vi "TSM Relay Connections to Configuration_v2.vi"(0 "TSM Context":T6, 5 "Relay/Action Connections":T4[](array[typedef]) {"Relay Action" items=["Open Relay"=20, "Close Relay"=21]}, 9 "TSM Site Numbers":i32[](array[numeric]), 11 "error in":errorcluster) -> (4 "TSM Relay Configuration":T1 {"SSC Relay with Action"."Relay Action" items=["Open Relay"=20, "Close Relay"=21]}, 15 "error out":errorcluster)   [LabVIEW 2019]
doc: "Populates the TSM Relay Configuration cluster for the selected relay/action connections. This VI can be used to implement a relay configuration (set of mappings between relays and positions) within a test code module. \n\nUse this VI in place of TSM Relay Conections to Configuration VI when optimizing for test time - this allows users to call Get Site Numbers only once in their code module and reduce the number of TSM context calls."
uses:
  <vilib>/NI_TestStand_SemiconductorModule/NI_TestStand_Semiconductor_Module.lvlibp/PinMap/General/SemiconductorModuleContext.ctl
  Pin Map/TSM Relay to Action Map.ctl
  <vilib>/NI_TestStand_SemiconductorModule/NI_TestStand_Semiconductor_Module.lvlibp/1abvi3w/instr.lib/niSwitch/niswitch.llb/niSwitch Relay Action.ctl
  SubVIs/TSM Relay Config.ctl
  <vilib>/NI_TestStand_SemiconductorModule/NI_TestStand_Semiconductor_Module.lvlibp/PinMap/PinQueryContext/MultiplePinMultipleSessionQueryContext/MultiplePinMultipleSessionQueryContext.lvclass
  SSC/SSC Relay.ctl
  <instrlib>/niSwitch/niSwitch.llb/niSwitch Relay Action.ctl
  <vilib>/NI_TestStand_SemiconductorModule/NI_TestStand_Semiconductor_Module.lvlibp
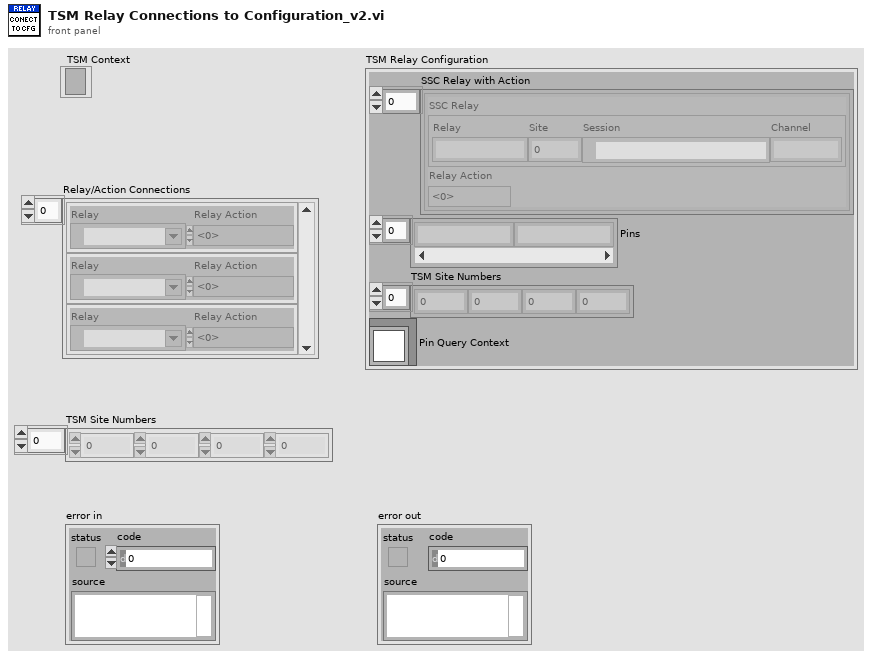
[diagram p1: front panel]
types:
  T1 = typedef "TSM Relay Config.ctl" = cluster{"SSC Relay with Action":cluster{"SSC Relay":T2, "Relay Action":T3}[], "Pins":string[], "TSM Site Numbers":i32[], "Pin Query Context":refnum<class "MultiplePinMultipleSessionQueryContext.lvclass">}
  T2 = typedef "SSC Relay.ctl" = cluster{"Relay":string, "Site":i32, "Session":refnum<k15>, "Channel":string}
  T3 = typedef "niSwitch Relay Action.ctl" = i32
  T4 = typedef "TSM Relay to Action Map.ctl" = cluster{"Relay":tag, "Relay Action":T5}
  T5 = typedef "NI_TestStand_Semiconductor_Module.lvlibp/niSwitch Relay Action.ctl" = i32
  T6 = typedef "NI_TestStand_Semiconductor_Module.lvlibp/SemiconductorModuleContext.ctl" = refnum<k7>
  T7 = typedef "TSM SSC Relay.ctl" = cluster{"TSM context":T6, "Pin Query Context":refnum<class "MultiplePinMultipleSessionQueryContext.lvclass">, "TSM Site Numbers":i32[], "SSC Relay":T2[], "Unfiltered Pins":string[], "Filtered Pins":string[], "Filtered Pins Info":T8}
  T8 = typedef "TSM Filtered Pins Info.ctl" = cluster{"Unfiltered Pins Count":i32, "Locations":i32[], "Lengths":i32[]}
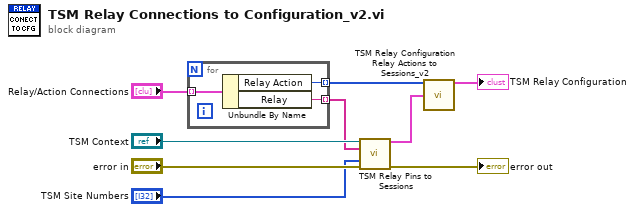
[diagram p0: block diagram]
diagram:
  n1 = for {
    tunnel: "Relay/Action Connections" -> [w11] mode=indexing
    tunnel: [w12] -> w2 mode=indexing
    tunnel: [w10] -> w5 mode=indexing
    n2 = Unbundle By Name(w11) -> ("Relay Action"=w10:T5, "Relay"=w12:tag)
  }
  n3 = call "TSM Relay Pins to Sessions.vi"("TSM context"="TSM Context", "Relay Pins"=w2, "Site Numbers"="TSM Site Numbers", "error in"="error in") -> ("TSM Relay"=w4:T7, "error out"=→"error out":errorcluster)  [unwired: 10 in]
  n4 = call "TSM Relay Configuration Relay Actions to Sessions_v2.vi"("Relay Actions"=w5, "TSM Relay In"=w4) -> ("TSM Relay Configuration Out"=→"TSM Relay Configuration":T1)  [unwired: 13 in]
